vi "KI6221.vi"() -> ()   [LabVIEW 2025] (continued)
                    n1511 = property on="Stop Level" class="DigNum (strict)"() -> ("Value"=w2022:dbl)  [unwired: 2 in, 2 out]
                    n1512 = while {
                      tunnel: w2020 -> [w2061]
                      shift-right: [w2068] -> _
                      shift-left: dbl[] [] -> [w2067]
                      tunnel: w2022 -> [w2066]
                      tunnel: w2008 -> [w2065]
                      i -> [w2058]
                      stop <- w2059 stop-if-true
                      n1513 = Subtract(x=w2065, y=1) -> (x-y=w2057:i32)
                      n1514 = Subtract(x=w2066, y=w2061) -> (x-y=w2063:dbl)
                      n1515 = Divide(x=w2063, y=w2057) -> (x/y=w2062:dbl)
                      n1516 = Multiply(x=w2062, y=w2058) -> (x*y=w2060:dbl)
                      n1517 = Add(x=w2061, y=w2060) -> (x+y=w2056:dbl)
                      n1518 = Insert Into Array(array=w2067, index=w2058, new element=w2056) -> (w2068:dbl[])
                      n1519 = Equal?(x=w2057, y=w2058) -> (x = y?=w2059:bool)
                    }
                    n1520 = while {
                      shift-right: [w2047] -> w2012
                      shift-left: w2011 -> [w2044]
                      shift-right: [w2046] -> w2013
                      shift-left: w2011 -> [w2043]
                      shift-right: [w2045] -> w2014
                      shift-left: w2011 -> [w2042]
                      tunnel: w2010 -> [w2040]
                      tunnel: [w2034] -> _
                      tunnel: w2004 -> [w2036]
                      tunnel: w2009 -> [w2035]
                      tunnel: w2008 -> [w2034]
                      i -> [w2038]
                      stop <- w2039 stop-if-true
                      n1521 = Multiply(x=6, y=w2038) -> (x*y=w2054:i32)
                      n1522 = Add(x=w2040, y=w2054) -> (x+y=w2053:i32)
                      n1523 = Add(x=w2035, y=w2054) -> (x+y=w2052:i32)
                      n1524 = Add(x=5, y=w2054) -> (x+y=w2051:i32)
                      n1525 = Index Array(array=w2036, index (col)=w2053) -> (element=w2050:string[])  [unwired: 1 in]
                      n1526 = Index Array(array=w2036, index (col)=w2052) -> (element=w2049:string[])  [unwired: 1 in]
                      n1527 = Index Array(array=w2036, index (col)=w2051) -> (element=w2048:string[])  [unwired: 1 in]
                      n1528 = Decrement(x=w2034) -> (x-1=w2037:i32)
                      n1529 = Build Array (concatenate)(w2044, w2050) -> (w2047:string[])
                      n1530 = Build Array (concatenate)(w2043, w2049) -> (w2046:string[])
                      n1531 = Build Array (concatenate)(w2042, w2048) -> (w2045:string[])
                      n1532 = Equal?(x=w2037, y=w2038) -> (x = y?=w2039:bool)
                    }
                    n1533 = call "Basic Properties.vi"("Differential Conductance Surface Plot"=w2015, "Int"=w2016, "fast draw"=TRUE) -> ("3D graph out"=w2007:refnum<k7>, "error out"=w2006:errorcluster)  [unwired: 11 in]
                    n1534 = Fract/Exp String To Number(string=w2012) -> (number=w1997:dbl[])  [unwired: 3 in, 1 out]
                    n1535 = To Variant(anything=w1997) -> (Variant=w1999:variant)
                    n1536 = Fract/Exp String To Number(string=w2013) -> (number=w1996:dbl[])  [unwired: 3 in, 1 out]
                    n1537 = To Variant(anything=w1996) -> (Variant=w1998:variant)
                    n1538 = Fract/Exp String To Number(string=w2014) -> (number=w2005:dbl[])  [unwired: 3 in, 1 out]
                    n1539 = To Variant(anything=w2005) -> (Variant=w2000:variant)
                    n1540 = call "Stub 3d Graph-3.vi"("3D graph out"=w2007, "Variant 3"=w2000, "Variant 2"=w1999, "error out 2"=w2006, "Variant"=w1998) -> ("error out"=→"error out 28":errorcluster)
                  }
                  frame True {
                  }
                }
                n1541 = case shown="True" "edit commands STEP SOURCE" {
                  frame False {
                  }
                  frame True {
                    # "HERE WE NEED TO SET THE STEP\nINPUTS TO THE INSTRUMENT \nCOMMANDS ON FILE FOR EDITING."
                    n1542 = property on="Select step source:" class="Ring (strict)"() -> ("Value"=w1987:u16)  [unwired: 2 in, 2 out]
                    n1543 = property on="MASTER DRIVER Array" class="Arr (strict)"() -> ("Value"=w1986:T9)  [unwired: 2 in, 2 out]
                    n1544 = property on="COMM\nTab Control" class="TabCtl (strict)"("Value"=T2."STEP CONFIG" ("COMM\nTab Control")) -> ()  [unwired: 2 in, 2 out]
                    n1545 = Index Array(array=w1986, index=w1987) -> (element=w1985:T14)
                    n1546 = property on="STEP EDIT VAR" class="Bool (strict)"("Value"=TRUE) -> ()  [unwired: 2 in, 2 out]
                    n1547 = Unbundle(w1985) -> ("Numeric"=w1984:i32, "String"=w1983:string, "String 2"=w1982:string, "String 3"=w1981:string, "String 4"=w1980:string, "String 5"=w1979:string, "String 6"=w1978:string, "Numeric 2"=w1977:i32)
                    n1548 = property on="GPIB Address:" class="DigNum (strict)"("Value"=w1984) -> ()  [unwired: 2 in, 2 out]
                    n1549 = property on="INSTRUMENT NAME:" class="Str"("Value"=w1983) -> ()  [unwired: 2 in, 2 out]
                    n1550 = property on="VERIFY:" class="Str"("Value"=w1982) -> ()  [unwired: 2 in, 2 out]
                    n1551 = property on="RESPONSE STRING:" class="Str"("Value"=w1981) -> ()  [unwired: 2 in, 2 out]
                    n1552 = local write "Main Tabs"(T1."General" ("Big Tabs")) -> ()
                    n1553 = property on="CONFIGURE:" class="Str"("Value"=w1980) -> ()  [unwired: 2 in, 2 out]
                    n1554 = property on="GO TO LEVEL:                *NOTE - MUST include <LEVEL>" class="Str"("Value"=w1979) -> ()  [unwired: 2 in, 2 out]
                    n1555 = property on="DEACTIVATE:" class="Str"("Value"=w1978) -> ()  [unwired: 2 in, 2 out]
                    n1556 = property on="DELAY in mS" class="DigNum (strict)"("Value"=w1977) -> ()  [unwired: 2 in, 2 out]
                  }
                }
                n1557 = case shown="True" "DELETE SOURCE" {
                  frame False {
                  }
                  frame True {
                    n1558 = property on="Select step source:" class="Ring (strict)"() -> ("Value"=w1972:u16, "Strings []"=w1974:string[])  [unwired: 2 in, 2 out]
                    n1559 = property on="MASTER DRIVER Array" class="Arr (strict)"() -> ("Value"=w1971:T9)  [unwired: 2 in, 2 out]
                    n1560 = Delete From Array(array=w1974, index=w1972) -> (array with subset deleted=w1975:string[])  [unwired: 1 in, 1 out]
                    n1561 = Decrement(x=w1972) -> (x-1=w1973:u16)
                    n1562 = property on="Select step source:" class="Ring (strict)"("Strings []"=w1975, "Value"=w1973) -> ()  [unwired: 2 in, 2 out]
                    n1563 = Delete From Array(array=w1971, index=w1972) -> (array with subset deleted=w1968:T9)  [unwired: 1 in, 1 out]
                    n1564 = property on="MASTER DRIVER Array" class="Arr (strict)"("Value"=w1968) -> ()  [unwired: 2 in, 2 out]
                    n1565 = property on="Default path" class="Path"() -> ("Value"=w1967:path)  [unwired: 2 in, 2 out]
                    n1566 = Build Path(base path=w1967, name or relative path="stepdriver.cfg" ("file path (dialog if empty)")) -> (appended path=w1965:path)
                    n1567 = Delete(path (use dialog)=w1965) -> (deleted path=w1969:path, error out=→"error out 11":errorcluster)  [unwired: 4 in, 1 out]
                    n1568 = Flatten To String(anything=w1968) -> (data string=w1970:string)  [unwired: 3 in, 2 out]
                    n1569 = call "WriteToFile.vi"("character string"=w1970, "file path (dialog if empty)"=w1969) -> ()  [unwired: 3 in, 1 out]
                  }
                }
                n1570 = property on="Select step source:" class="Ring (strict)"() -> ("Strings []"=w1862:string[])  [unwired: 2 in, 2 out]
                n1571 = Array Size(array=w1862) -> (size(s)=w1861:i32)
                n1572 = Not Equal?(x="Select step source:", y="STEP SOURCE LAST") -> (x != y?=w1855:bool)
                n1573 = Decrement(x=w1861) -> (x-1=w1860:i32)
                n1574 = Equal?(x="Select step source:", y=w1860) -> (x = y?=w1857:bool)
                n1575 = Not(x=w1857) -> (.not. x?=w1856:bool)
                n1576 = And(x=w1856, y=w1855) -> (x .and. y?=w1863:bool)
                n1577 = case shown="True" w1863 {
                  tunnel: "Select step source:" -> [_ w1953]
                  frame False {
                  }
                  frame True {
                    n1578 = property on="MASTER DRIVER Array" class="Arr (strict)"() -> ("Value"=w1954:T9)  [unwired: 2 in, 2 out]
                    n1579 = property on="STEP SOURCE LAST" class="DigNum (strict)"("Value"=w1953) -> ()  [unwired: 2 in, 2 out]
                    n1580 = Index Array(array=w1954, index=w1953) -> (element=w1955:T14)
                    n1581 = Unbundle(w1955) -> ("Numeric"=w1956:i32, "String"=w1957:string, "String 2"=w1958:string, "String 3"=w1959:string, "String 4"=w1960:string, "String 5"=w1961:string, "String 6"=w1962:string, "Numeric 2"=w1963:i32)
                    n1582 = property on="GPIB Address:" class="DigNum (strict)"("Value"=w1956) -> ()  [unwired: 2 in, 2 out]
                    n1583 = property on="INSTRUMENT NAME:" class="Str"("Value"=w1957) -> ()  [unwired: 2 in, 2 out]
                    n1584 = property on="VERIFY:" class="Str"("Value"=w1958) -> ()  [unwired: 2 in, 2 out]
                    n1585 = property on="RESPONSE STRING:" class="Str"("Value"=w1959) -> ()  [unwired: 2 in, 2 out]
                    n1586 = property on="CONFIGURE:" class="Str"("Value"=w1960) -> ()  [unwired: 2 in, 2 out]
                    n1587 = property on="GO TO LEVEL:                *NOTE - MUST include <LEVEL>" class="Str"("Value"=w1961) -> ()  [unwired: 2 in, 2 out]
                    n1588 = property on="DEACTIVATE:" class="Str"("Value"=w1962) -> ()  [unwired: 2 in, 2 out]
                    n1589 = property on="DELAY in mS" class="DigNum (strict)"("Value"=w1963) -> ()  [unwired: 2 in, 2 out]
                  }
                }
                n1590 = case shown="True" w1857 {
                  frame False {
                  }
                  frame True {
                    w1992 = ""
                    w1993 = 20
                    n1591 = property on="STEP EDIT VAR" class="Bool (strict)"("Value"=FALSE ("Visible")) -> ()  [unwired: 2 in, 2 out]
                    n1592 = local write "Main Tabs"(T1."General" ("Big Tabs")) -> ()
                    n1593 = property on="COMM\nTab Control" class="TabCtl (strict)"("Value"=T2."STEP CONFIG" ("COMM\nTab Control")) -> ()  [unwired: 2 in, 2 out]
                    n1594 = property on="GPIB Address:" class="DigNum (strict)"("Value"=w1993) -> ()  [unwired: 2 in, 2 out]
                    n1595 = property on="INSTRUMENT NAME:" class="Str"("Value"=w1992) -> ()  [unwired: 2 in, 2 out]
                    n1596 = property on="VERIFY:" class="Str"("Value"=w1992) -> ()  [unwired: 2 in, 2 out]
                    n1597 = property on="RESPONSE STRING:" class="Str"("Value"=w1992) -> ()  [unwired: 2 in, 2 out]
                    n1598 = property on="CONFIGURE:" class="Str"("Value"=w1992) -> ()  [unwired: 2 in, 2 out]
                    n1599 = property on="GO TO LEVEL:                *NOTE - MUST include <LEVEL>" class="Str"("Value"=w1992) -> ()  [unwired: 2 in, 2 out]
                    n1600 = property on="DEACTIVATE:" class="Str"("Value"=w1992) -> ()  [unwired: 2 in, 2 out]
                    n1601 = property on="DELAY in mS" class="DigNum (strict)"("Value"=w1993) -> ()  [unwired: 2 in, 2 out]
                  }
                }
                n1602 = case shown="0, Default" "I want to control my test in terms of:" {
                  frame 0, Default {
                    w1909 = 105.0 ("y")
                    w1896 = 2
                    # "overlimit\nmultiplier"
                    n1603 = local read "Number of sweep points"() -> (w1914:i32)
                    n1604 = local read "Start Voltage  (Volts)"() -> (w1918:dbl)
                    n1605 = Absolute Value(x=w1918) -> (abs(x)=w1897:dbl)
                    n1606 = local read "Stop Voltage (Volts)"() -> (w1917:dbl)
                    n1607 = Absolute Value(x=w1917) -> (abs(x)=w1898:dbl)
                    n1608 = Greater?(x=w1897, y=w1898) -> (0:w1920:bool)
                    n1609 = Select(t=w1897, s=w1920, f=w1898) -> (s? t:f=w1919:dbl)
                    n1610 = Subtract(x=w1918, y=w1917) -> (x-y=w1915:dbl)
                    n1611 = Absolute Value(x=w1919) -> (abs(x)=w1911:dbl)
                    n1612 = Absolute Value(x=w1915) -> (abs(x)=w1910:dbl)
                    n1613 = Divide(x=w1910, y=w1914) -> (x/y=w1916:dbl)
                    n1614 = Add(x=w1911, y=w1916) -> (x+y=w1913:dbl)
                    n1615 = Multiply(x=w1913, y=1.15) -> (x*y=w1905:dbl)
                    n1616 = Greater?(x=w1905, y=w1909) -> (0:w1908:bool)
                    n1617 = Greater?(x=w1905, y=12.0) -> (0:w1906:bool)
                    n1618 = case shown="False" w1906 {
                      tunnel: [w1934 100.0 ("y")] -> w1899
                      tunnel: w1905 -> [w1933 _]
                      frame False {
                        n1619 = Greater?(x=w1933, y=1.2) -> (0:w1935:bool)
                        n1620 = case shown="False" w1935 {
                          tunnel: [w1938 10.0 ("y")] -> w1934
                          tunnel: w1933 -> [w1937 _]
                          frame False {
                            n1621 = Greater?(x=w1937, y=0.12) -> (0:w1939:bool)
                            n1622 = case shown="False" w1939 {
                              tunnel: [w1942 1.0 ("y")] -> w1938
                              tunnel: w1937 -> [w1941 _]
                              frame False {
                                n1623 = Greater?(x=w1941, y=0.012) -> (0:w1943:bool)
                                n1624 = case shown="False" w1943 {
                                tunnel: [0.01 0.1 ("y")] -> w1942
                                frame False {
                                }
                                frame True {
                                }
                                }
                              }
                              frame True {
                              }
                            }
                          }
                          frame True {
                          }
                        }
                      }
                      frame True {
                      }
                    }
                    n1625 = property on="Voltage Measure Range" class="Ring (strict)"("Disabled"=w1896, "Value"=w1899) -> ()  [unwired: 2 in, 2 out]
                    n1626 = case shown="False" w1908 {
                      tunnel: w1909 -> [_ w1951]
                      tunnel: [w1950 w1951] -> w1904
                      tunnel: w1905 -> [w1950 _]
                      frame False {
                      }
                      frame True {
                      }
                    }
                    n1627 = case shown="False" "Case Constant\n(See Context Help) 5" {
                      tunnel: w1904 -> [w1928 w1932]
                      tunnel: [w1922 w1931] -> w1902
                      frame False {
                        w1921 = 0.1 ("y")
                        w1925 = 100.0 ("y")
                        n1628 = Multiply(x=w1928, y=w1925) -> (x*y=w1927:dbl)
                        n1629 = Round Toward +Infinity(x=w1927) -> (ceil(x): smallest int >= x=w1926:dbl)
                        n1630 = Divide(x=w1926, y=w1925) -> (x/y=w1923:dbl)
                        n1631 = Greater?(x=w1923, y=w1921) -> (0:w1924:bool)
                        n1632 = case shown="False" w1924 {
                          tunnel: [w1929 w1930] -> w1922
                          tunnel: w1923 -> [_ w1930]
                          tunnel: w1921 -> [w1929 _]
                          frame False {
                          }
                          frame True {
                          }
                        }
                      }
                      frame True {
                        n1633 = Round Toward +Infinity(x=w1932) -> (ceil(x): smallest int >= x=w1931:dbl)
                      }
                    }
                    n1634 = Multiply(x=w1902, y=1.2) -> (x*y=w1901:dbl)
                    n1635 = property on="Current Source \nVoltage Compliance (V)" class="DigNum (strict)"("Disabled"=w1896, "Value"=w1901) -> ()  [unwired: 2 in, 2 out]
                  }
                  frame 1 {
                    w1952 = u8 0 ("Disabled")
                    n1636 = property on="Current Source \nVoltage Compliance (V)" class="DigNum (strict)"("Disabled"=w1952) -> ()  [unwired: 2 in, 2 out]
                    n1637 = property on="Voltage Measure Range" class="Ring (strict)"("Disabled"=w1952) -> ()  [unwired: 2 in, 2 out]
                  }
                }
              }
              frame "Pulsed IV Measurements" {
                # "Fliter visible..."
                # "PULSE CONTROLS NOT DIRECTLY LINKED."
                # "CLEAR DATA from sheet and graph"
                # "SAVE DATA to file"
                # "Update Pulse TABS"
                # "UPDATE GRAPH AXIS WHEN SELECTIONS ARE CHANGED"
                # "ENABLE PULSE COUNT ON INF OFF SETTING"
                n1638 = case shown="0, Default" "Pulse Mode:" {
                  tunnel: [enum32{"DIAGRAM 2", "DIAGRAM"}."DIAGRAM 2" ("PULSE HELP TABS") enum32{"DIAGRAM 2", "DIAGRAM"}."DIAGRAM" ("PULSE HELP TABS")] -> w3061
                  frame 0, Default {
                  }
                  frame 1 {
                  }
                }
                n1639 = local write "PULSE SWEEP OR LEVEL TABS"("Pulse Mode:") -> ()
                n1640 = Boolean To (0,1)(Boolean="INFINITE REPEAT PULSE CYCLES") -> (0, 1=w3077:i16)
                n1641 = Multiply(x=w3077, y=i16 2) -> (x*y=w3076:i16)
                n1642 = property on="Number of Readings" class="DigNum (strict)"("Disabled"=w3076) -> ()  [unwired: 2 in, 2 out]
                n1643 = local write "PULSE HELP TABS"(w3061) -> ()
                n1644 = case shown="True" "PULSE SAVE DATA" {
                  frame False {
                  }
                  frame True {
                    n1645 = File Dialog(4:"KI Data files" ("pattern label"), 5:"Save As" ("button label"), 6:"*.kdf" ("pattern label")) -> (1:w3633:bool, 3:w3632:path)  [unwired: 4 in, 2 out]
                    n1646 = case shown="False" w3633 {
                      tunnel: w3632 -> [w3637 _]
                      frame False {
                        w3641 = "%s" ("format string")
                        n1647 = property on="PULSE DATA SHEET" class="Tbl (strict)"() -> ("Column Header Strings[]"=w3642:string[], "Value"=w3643:string[][])  [unwired: 2 in, 2 out]
                        n1648 = Array To Spreadsheet String(array=w3643, 3:w3641) -> (spreadsheet string=w3639:string)  [unwired: 1 in]
                        n1649 = Array To Spreadsheet String(array=w3642, 3:w3641) -> (spreadsheet string=w3640:string)  [unwired: 1 in]
                        n1650 = Concatenate Strings(w3640, w3639) -> (w3638:string)
                        n1651 = call "WriteToFile.vi"("character string"=w3638, "file path (dialog if empty)"=w3637) -> ()  [unwired: 3 in, 1 out]
                      }
                      frame True {
                      }
                    }
                  }
                }
                n1652 = case shown="True" "RUN PULSE" {
                  frame False {
                  }
                  frame True {
                    w3103 = FALSE
                    w3101 = TRUE
                    w3130 = "%s" ("format string")
                    w3111 = 0
                    w3113 = u16 2 ("x")
                    # "SETUP FOR TEST RUN. INIT controls."
                    # "RESET ENABLES FOR \nNEW TEST RUN."
                    n1653 = property on="ABORT PULSE" class="Bool (strict)"("Value"=FALSE, "Disabled"=u16 0 ("x")) -> (error out=w3137:errorcluster)  [unwired: 2 in, 1 out]
                    n1654 = property on="Main Tabs" class="TabCtl (strict)"("Page Selector Visible"=w3103) -> (error out=w3104:errorcluster)  [unwired: 2 in, 1 out]
                    n1655 = property on="Advanced Operation Tab" class="TabCtl (strict)"(error in=w3104, "Page Selector Visible"=w3103) -> (error out=w3114:errorcluster)  [unwired: 1 in, 1 out]
                    n1656 = local read "Current Test File:"() -> (w3105:path)
                    n1657 = Equal?(x=w3105, y=path "") -> (x = y?=w3119:bool)
                    n1658 = case shown="True" w3119 {
                      tunnel: w3105 -> [w3151 _]
                      tunnel: [w3146 w3152] -> w3118
                      frame False {
                        n1659 = Path To String(path=w3151) -> (string=w3149:string)
                        n1660 = Search/Split String(string=w3149, search string/char (-)=".") -> (substring before match=w3148:string)  [unwired: 1 in, 2 out]
                        n1661 = Concatenate Strings(w3148, "_pulsedata.kdf" ("search string/char (-)")) -> (w3145:string)
                        n1662 = String To Path(string=w3145) -> (path=w3146:path)
                      }
                      frame True {
                        n1663 = property on="Default path" class="Path"() -> ("Value"=w3154:path)  [unwired: 2 in, 2 out]
                        n1664 = Build Path(base path=w3154, name or relative path="DefaultTestFile_pulsedata.cfg" ("file path (dialog if empty)")) -> (appended path=w3152:path)
                      }
                    }
                    n1665 = property on="RUN PULSE" class="Bool"(error in=w3114, "Disabled"=w3113) -> (error out=w3116:errorcluster)  [unwired: 1 in, 1 out]
                    n1666 = invoke on="PULSE DATA SHEET" class="Table" method="Reinit To Default"(error in=w3116) -> (error out=w3108:errorcluster)  [unwired: 2 in, 2 out]
                    n1667 = invoke on="Pulsed IV Graph" class="XYGraph (strict)" method="Reinit To Default"(error in=w3108) -> (error out=w3107:errorcluster)  [unwired: 2 in, 2 out]
                    n1668 = property on="DEMO MODE" class="Bool (strict)"(error in=w3107) -> ("Value"=w3144:bool)  [unwired: 1 in, 2 out]
                    n1669 = property on="X Axis:" class="Ring (strict)"("Disabled"=w3113) -> ("Value"=w3140:u16, "Strings []"=w3143:string[])  [unwired: 2 in, 2 out]
                    n1670 = Index Array(array=w3143, index=w3140) -> (element=w3110:string)
                    n1671 = property on="Y Axis:" class="Ring (strict)"("Disabled"=w3113) -> ("Value"=w3141:u16, "Strings []"=w3142:string[])  [unwired: 2 in, 2 out]
                    n1672 = call <vilib>:"Read Lines From File.vi"("convert eol? (no:F)"=TRUE, "file path (dialog if empty)"=w3118, "number of lines (all:-1)"=-1) -> ("line string"=w3128:string)  [unwired: 3 in, 3 out]
                    n1673 = Match Pattern(string=w3128, regular expression="\n") -> (before substring=w3126:string, match substring=w3125:string, after substring=w3123:string)  [unwired: 1 in, 1 out]
                    n1674 = Index Array(array=w3142, index=w3141) -> (element=w3109:string)
                    n1675 = property on="Pulsed IV Graph" class="XYGraph (strict)"("X Scale.Name Label.Text"=w3110, "Y Scale.Name Label.Text"=w3109) -> ()  [unwired: 2 in, 2 out]
                    n1676 = Concatenate Strings(w3126, w3125) -> (w3124:string)
                    n1677 = Spreadsheet String To Array(format string=w3130, spreadsheet string=w3123, array type (2D Dbl)=string[][] []) -> (array=w3117:string[][])  [unwired: 1 in]
                    n1678 = Spreadsheet String To Array(format string=w3130, spreadsheet string=w3124, array type (2D Dbl)=string[] []) -> ()  [unwired: 1 in, 1 out]
                    n1679 = case shown="False" w3144 {
                      tunnel: w3117 -> [_ w3590]
                      tunnel: w3141 -> [_ w3588]
                      tunnel: w3140 -> [_ w3589]
                      tunnel: w3137 -> [w3176 w3596]
                      tunnel: [w3176 w3596] -> w3136
                      tunnel: [w3175 w3587] -> w3133
                      frame False {
                        # "PULSE MODE CONTROL\nCHECKS - OK TO \nCONTINUE WITH RUN?"
                        n1680 = property on="Select the nanovoltmeter model number:" class="Ring (strict)"() -> ("Value"=w3181:u16)  [unwired: 2 in, 2 out]
                        n1681 = property on="Start Pulse Level (Amps)" class="DigNum (strict)"() -> ("Value"=w3191:dbl)  [unwired: 2 in, 2 out]
                        n1682 = property on="Stop Pulse Level (Amps)" class="DigNum (strict)"() -> ("Value"=w3190:dbl)  [unwired: 2 in, 2 out]
                        n1683 = property on="Pulse Mode:" class="Ring (strict)"() -> ("Value"=w3192:u16)  [unwired: 2 in, 2 out]
                        n1684 = property on="Sweep Type" class="Ring (strict)"() -> ("Value"=w3185:u16)  [unwired: 2 in, 2 out]
                        n1685 = property on="Select the current source model number:" class="Ring (strict)"() -> ("Value"=w3174:u16)  [unwired: 2 in, 2 out]
                        n1686 = Equal?(x=w3181, y=3) -> (x = y?=w3178:bool)
                        n1687 = Equal?(x=w3174, y=2) -> (x = y?=w3155:bool)
                        n1688 = property on="Pulse Width (mS)" class="DigNum (strict)"() -> ("Value"=w3173:dbl)  [unwired: 2 in, 2 out]
                        n1689 = Not Equal To 0?(x=w3192) -> (x != 0?=w3186:bool)
                        n1690 = Greater Than 0?(x=w3191) -> (x > 0?=w3189:bool)
                        n1691 = property on="Delay - pulse settle time in mS" class="DigNum (strict)"() -> ("Value"=w3159:dbl)  [unwired: 2 in, 2 out]
                        n1692 = Less?(x=w3159, y=0.5) -> (x < y?=w3168:bool)
                        n1693 = And(x=w3178, y=w3155) -> (x .and. y?=w3177:bool)
                        n1694 = Equal To 0?(x=w3185) -> (x = 0?=w3184:bool)
                        n1695 = Less?(x=w3159, y=0.055) -> (x < y?=w3164:bool)
                        n1696 = Greater Than 0?(x=w3190) -> (x > 0?=w3188:bool)
                        n1697 = And(x=w3189, y=w3188) -> (x .and. y?=w3187:bool)
                        n1698 = property on="Voltage Measure Range" class="Ring (strict)"() -> ("Value"=w3156:dbl)  [unwired: 2 in, 2 out]
                        n1699 = Equal?(x=100.0, y=w3156) -> (x = y?=w3166:bool)
                        n1700 = And(x=w3168, y=w3166) -> (x .and. y?=w3169:bool)
                        n1701 = Add(x=0.034, y=w3159) -> (x+y=w3171:dbl)
                        n1702 = Greater Or Equal?(x=w3173, y=w3171) -> (x >= y?=w3172:bool)
                        n1703 = Compound Arithmetic op=OR(w3186, w3187, w3184) -> (w3182:bool)
                        n1704 = Equal?(x=0.01, y=w3156) -> (x = y?=w3162:bool)
                        n1705 = And(x=w3164, y=w3162) -> (x .and. y?=w3160:bool)
                        n1706 = Or(x=w3169, y=w3160) -> (x .or. y?=w3158:bool)
                        n1707 = case shown="True" w3158 {
                          tunnel: [TRUE ("OK") w3194] -> w3157
                          frame False {
                          }
                          frame True {
                            # "SEND WARNING"
                            n1708 = call "Pulse delay warning"() -> ("OK"=w3194:bool)  [unwired: 10 in, 1 out]
                          }
                        }
                        n1709 = Compound Arithmetic op=AND(w3182, w3177, w3172, w3157) -> (w3183:bool)
                        n1710 = case shown="False" w3183 {
                          tunnel: w3182 -> [w3198 _]
                          tunnel: w3177 -> [w3197 _]
                          tunnel: [FALSE w3209] -> w3175
                          tunnel: w3172 -> [w3195 _]
                          tunnel: w3156 -> [_ w3208]
                          frame False {
                            n1711 = case shown="False" w3195 {
                              frame False {
                                n1712 = One Button Dialog(message="For Pulsed IV measurements the pulse width must be greater than or equal to\nthe delay (settling time) plus 34 us for the measurement. Please correct the settings.") -> (true=w3199:bool)  [unwired: 1 in]
                                n1713 = case shown="False" w3199 {
                                frame False {
                                }
                                frame True, Default {
                                n1714 = property on="Delay - pulse settle time in mS" class="DigNum (strict)"("Key Focus"=TRUE) -> ()  [unwired: 2 in, 2 out]
                                }
                                }
                              }
                              frame True {
                              }
                            }
                            n1715 = case shown="False" w3197 {
                              frame False {
                                n1716 = One Button Dialog(message="Taking pulsed IV measurements requires both a Model 6221 current\nsource and a Model 2182A nanovoltmeter connected to the bus and \nconfigured in the instrument communication panel.") -> (true=w3202:bool)  [unwired: 1 in]
                                n1717 = case shown="False" w3202 {
                                frame False {
                                }
                                frame True, Default {
                                }
                                }
                              }
                              frame True {
                              }
                            }
                            n1718 = case shown="False" w3198 {
                              frame False {
                                n1719 = One Button Dialog(message="To run a test with a logarithmic pulse sweep, both start and stop\npulse values must be positive. Change a value, then click RUN again.") -> (true=w3204:bool)  [unwired: 1 in]
                                n1720 = case shown="True" w3204 {
                                frame False {
                                }
                                frame True, Default {
                                n1721 = property on="Start Pulse Level (Amps)" class="DigNum (strict)"("Key Focus"=TRUE) -> ()  [unwired: 2 in, 2 out]
                                }
                                }
                              }
                              frame True {
                              }
                            }
                          }
                          frame True {
                            (unwired) "Initiating Test. Make certain device is correctly connected\nto the instruments, then click OK. "
                            # "ACTUAL DATA \nCOMMUNICATION"
                            n1722 = property on="X Axis:" class="Ring (strict)"() -> ("Value"=w3211:u16)  [unwired: 2 in, 2 out]
                            n1723 = property on="Y Axis:" class="Ring (strict)"() -> ("Value"=w3210:u16)  [unwired: 2 in, 2 out]
                            n1724 = case shown="True" "Case Constant\n(See Context Help) 6" {
                              tunnel: [FALSE w3219] -> w3209
                              tunnel: w3211 -> [_ w3223]
                              tunnel: w3210 -> [_ w3222]
                              tunnel: w3208 -> [_ w3220]
                              frame False {
                              }
                              frame True {
                                # "TEST MODEL NUMBER AT VISA \nRESOURCE..."
                                # "no NV"
                                # "NOT 6221"
                                n1725 = property on="6220 VISA" class="VISAName"() -> ("Value"=w3218:refnum<visa-resource-name>)  [unwired: 2 in, 2 out]
                                n1726 = property on="GPIB Array" class="Arr (strict)"() -> ("Value"=w3217:string[])  [unwired: 2 in, 2 out]
                                n1727 = call "VISAreadWrite.vi"("GPIB INDEX Array"=i32[] [0, 14], "GPIB ARRAY"=w3217, "VISA REFERENCE"=w3218) -> ("error out 15"=→"error out 17":errorcluster, "Read Buffer Array"=w3229:string[])  [unwired: 1 in]
                                n1728 = Index Array(array=w3229, index=1) -> (element=w3234:string)
                                n1729 = Match Pattern(string=w3234, regular expression="MODEL 6221") -> (offset past match=w3226:i32)  [unwired: 1 in, 3 out]
                                n1730 = Equal?(x=w3226, y=-1) -> (x = y?=w3224:bool)
                                n1731 = Index Array(array=w3229, index=5) -> (element=w3228:string)
                                n1732 = Decimal String To Number(string=w3228) -> (number=w3227:i32)  [unwired: 2 in, 1 out]
                                n1733 = Equal To 0?(x=w3227) -> (x = 0?=w3225:bool)
                                n1734 = Or(x=w3225, y=w3224) -> (x .or. y?=w3214:bool)
                                n1735 = case shown="False" w3214 {
                                tunnel: w3225 -> [_ w3585]
                                tunnel: w3224 -> [_ w3583]
                                tunnel: w3217 -> [w3361 _]
                                tunnel: w3218 -> [w3315 _]
                                tunnel: w3223 -> [w3310 _]
                                tunnel: w3222 -> [w3338 _]
                                tunnel: w3220 -> [w3296 _]
                                tunnel: [TRUE FALSE] -> w3213
                                frame False {
                                # "SWEEP RANGE FOR LOG - AUTO\ndc SWEEPS TOO.\nif off value < 2% of Max current value of pulse \nOR < 4 pA then do power..."
                                # "special pulse sweep delay fix\nround(NPLC*INC-6)/1000 = delay"
                                # "type"
                                # "count"
                                # "state"
                                # "TEST FOR ALL ZERO\nMEASUREMENTS FROM\nRANGE ERROR - DISP\nMessage..."
                                # "UPDATE SCPI STRINGS THEN LOAD THEM TO THE INSTRUMENT."
                                # "CREATE SCPI STRINGS FROM CONTROLS"
                                # "Check for data in buffer... when you get some, place it in data sheet and graph. REPEAT until all data is collected."
                                # "FIX SOURCE CURRENT"
                                n1736 = property on="Pulse Mode:" class="Ring (strict)"() -> ("Value"=w3264:u16)  [unwired: 2 in, 2 out]
                                n1737 = property on="Interval between Pulses (NPLC)" class="DigNum (strict)"() -> ("Value"=w3272:dbl)  [unwired: 2 in, 2 out]
                                n1738 = property on="Pulse Width (mS)" class="DigNum (strict)"() -> ("Value"=w3302:dbl)  [unwired: 2 in, 2 out]
                                n1739 = Not Equal To 0?(x="PULSE FILTER") -> (x != 0?=w3286:bool)
                                n1740 = property on="Number of Readings" class="DigNum (strict)"() -> ("Value"=w3321:i32)  [unwired: 2 in, 2 out]
                                n1741 = property on="INFINITE REPEAT PULSE CYCLES" class="Bool (strict)"() -> ("Value"=w3360:bool)  [unwired: 2 in, 2 out]
                                n1742 = local read "Pulse Filter Count"() -> (w3292:i32)
                                n1743 = case shown="2" "PULSE FILTER" {
                                tunnel: ["MOV" "MOV" "REP"] -> w3291
                                frame 0, Default {
                                }
                                frame 1 {
                                }
                                frame 2 {
                                }
                                }
                                n1744 = property on="Start Pulse Level (Amps)" class="DigNum (strict)"() -> ("Value"=w3263:dbl)  [unwired: 2 in, 2 out]
                                n1745 = property on="Stop Pulse Level (Amps)" class="DigNum (strict)"() -> ("Value"=w3262:dbl)  [unwired: 2 in, 2 out]
                                n1746 = property on="Pulse Level (Amps)" class="DigNum (strict)"() -> ("Value"=w3261:dbl)  [unwired: 2 in, 2 out]
                                n1747 = property on="Number of Pulses" class="DigNum (strict)"() -> ("Value"=w3319:i32)  [unwired: 2 in, 2 out]
                                n1748 = property on="Sweep Type" class="Ring (strict)"() -> ("Value"=w3249:u16)  [unwired: 2 in, 2 out]
                                n1749 = Equal?(x=w3249, y=u16 1) -> (x = y?=w3285:bool)
                                n1750 = property on="Pulse Off Level (Amps)" class="DigNum (strict)"() -> ("Value"=w3256:dbl)  [unwired: 2 in, 2 out]
                                n1751 = And(x=w3286, y=w3285) -> (x .and. y?=w3284:bool)
                                n1752 = property on="Delay - pulse settle time in mS" class="DigNum (strict)"() -> ("Value"=w3304:dbl)  [unwired: 2 in, 2 out]
                                n1753 = case shown="False" w3284 {
                                tunnel: ["0" "1"] -> w3289
                                frame False {
                                }
                                frame True {
                                }
                                }
                                n1754 = Number To Decimal String(number=w3272) -> (decimal integer string=w3346:string)  [unwired: 1 in]
                                n1755 = Negate(x=w3256) -> (-x=w3330:dbl)
                                n1756 = Divide(x=w3302, y=1000.0) -> (x/y=w3301:dbl)
                                n1757 = Divide(x=w3304, y=1000.0) -> (x/y=w3300:dbl)
                                n1758 = Number To Decimal String(number=w3292) -> (decimal integer string=w3290:string)  [unwired: 1 in]
                                n1759 = Number To Exponential String(number=w3261) -> (E-format string=w3349:string)  [unwired: 3 in]
                                n1760 = case shown="1" w3264 {
                                tunnel: ["1" "0"] -> w3329
                                tunnel: w3321 -> [_ w3576]
                                tunnel: [w3574 w3576] -> w3320
                                tunnel: w3319 -> [w3574 _]
                                frame 0, Default {
                                }
                                frame 1 {
                                }
                                }
                                n1761 = Equal?(x=w3330, y=w3261) -> (x = y?=w3316:bool)
                                n1762 = property on="Current Source \nVoltage Compliance (V)" class="DigNum (strict)"() -> ("Value"=w3340:dbl)  [unwired: 2 in, 2 out]
                                n1763 = Number To Exponential String(number=w3256) -> (E-format string=w3348:string)  [unwired: 3 in]
                                n1764 = Number To Exponential String(number=w3301) -> (E-format string=w3345:string)  [unwired: 3 in]
                                n1765 = Number To Exponential String(number=w3300) -> (E-format string=w3343:string)  [unwired: 3 in]
                                n1766 = Number To Exponential String(number=w3340) -> (E-format string=w3328:string)  [unwired: 3 in]
                                n1767 = case shown="1" w3249 {
                                tunnel: ["BEST" "AUTO"] -> w3248
                                frame 0, Default {
                                }
                                frame 1 {
                                }
                                }
                                n1768 = Decrement(x=w3319) -> (x-1=w3318:i32)
                                n1769 = case shown="False" w3360 {
                                tunnel: [w3579 "INF"] -> w3347
                                tunnel: w3320 -> [w3578 _]
                                tunnel: [w3578 0 ("Value")] -> w3311
                                frame False {
                                n1770 = Number To Decimal String(number=w3578) -> (decimal integer string=w3579:string)  [unwired: 1 in]
                                }
                                frame True {
                                }
                                }
                                n1771 = local read "INCREMENT"() -> (w3271:dbl)
                                n1772 = Multiply(x=w3272, y=w3271) -> (x*y=w3279:dbl)
                                n1773 = Divide(x=w3302, y=w3279) -> (x/y=w3305:dbl)
                                n1774 = case shown="1" w3249 {
                                tunnel: ["LIN" "LOG"] -> w3323
                                frame 0, Default {
                                }
                                frame 1 {
                                }
                                }
                                n1775 = Number To Exponential String(number=w3296) -> (E-format string=w3344:string)  [unwired: 3 in]
                                n1776 = Number To Decimal String(number="Number of Pulse Off Measurements") -> (decimal integer string=w3276:string)  [unwired: 1 in]
                                n1777 = Number To Exponential String(number=w3263) -> (E-format string=w3327:string)  [unwired: 3 in]
                                n1778 = Number To Exponential String(number=w3262) -> (E-format string=w3326:string)  [unwired: 3 in]
                                n1779 = Subtract(x=w3262, y=w3263) -> (x-y=w3322:dbl)
                                n1780 = Multiply(x=w3272, y=w3271) -> (x*y=w3270:dbl)
                                n1781 = Divide(x=w3322, y=w3318) -> (x/y=w3274:dbl)
                                n1782 = Number To Exponential String(number=w3274) -> (E-format string=w3325:string)  [unwired: 3 in]
                                n1783 = Subtract(x=w3270, y=6.0) -> (x-y=w3268:dbl)
                                n1784 = Round To Nearest(number=w3268) -> (nearest integer value=w3246:dbl)
                                n1785 = Insert Into Array(array=string[] [] ("Replace Array"), new element=w3349) -> (w3358:string[])  [unwired: 1 in]
                                n1786 = Equal?(x=w3246, y=77.0) -> (x = y?=w3247:bool)
                                n1787 = Insert Into Array(array=w3358, new element=w3348) -> (w3357:string[])  [unwired: 1 in]
                                n1788 = case shown="0, Default" w3264 {
                                tunnel: w3263 -> [w3372 _]
                                tunnel: w3262 -> [w3371 _]
                                tunnel: w3261 -> [_ w3374]
                                tunnel: [w3367 w3373] -> w3254
                                frame 0, Default {
                                n1789 = Absolute Value(x=w3372) -> (abs(x)=w3370:dbl)
                                n1790 = Absolute Value(x=w3371) -> (abs(x)=w3369:dbl)
                                n1791 = Greater?(x=w3370, y=w3369) -> (0:w3368:bool)
                                n1792 = Select(t=w3370, s=w3368, f=w3369) -> (s? t:f=w3367:dbl)
                                }
                                frame 1 {
                                n1793 = Absolute Value(x=w3374) -> (abs(x)=w3373:dbl)
                                }
                                }
                                n1794 = case shown="True" w3247 {
                                tunnel: w3246 -> [w3363 _]
                                tunnel: [w3363 1.0] -> w3244
                                frame False {
                                }
                                frame True {
                                }
                                }
                                n1795 = Insert Into Array(array=w3357, new element=w3347) -> (w3356:string[])  [unwired: 1 in]
                                n1796 = Insert Into Array(array=w3356, new element=w3327) -> (w3355:string[])  [unwired: 1 in]
                                n1797 = Insert Into Array(array=w3355, new element=w3346) -> (w3354:string[])  [unwired: 1 in]
                                n1798 = Insert Into Array(array=w3354, new element=w3345) -> (w3341:string[])  [unwired: 1 in]
                                n1799 = Insert Into Array(array=w3341, new element=w3328) -> (w3353:string[])  [unwired: 1 in]
                                n1800 = Insert Into Array(array=w3353, new element=w3344) -> (w3352:string[])  [unwired: 1 in]
                                n1801 = Insert Into Array(array=w3352, new element=w3343) -> (w3351:string[])  [unwired: 1 in]
                                n1802 = Insert Into Array(array=w3351, new element=w3329) -> (w3350:string[])  [unwired: 1 in]
                                n1803 = Insert Into Array(array=w3350, new element=w3325) -> (w3339:string[])  [unwired: 1 in]
                                n1804 = Insert Into Array(array=w3339, new element=w3326) -> (w3324:string[])  [unwired: 1 in]
                                n1805 = local read "Setup String"() -> (w3298:string)
                                n1806 = Add(x=u16 3, y=w3338) -> (x+y=w3308:u16)
                                n1807 = Divide(x=w3244, y=1000.0) -> (x/y=w3266:dbl)
                                n1808 = Insert Into Array(array=w3324, new element=w3323) -> (w3297:string[])  [unwired: 1 in]
                                n1809 = Number To Exponential String(number=w3266) -> (E-format string=w3265:string)  [unwired: 3 in]
                                n1810 = Absolute Value(x=w3256) -> (abs(x)=w3252:dbl)
                                n1811 = Less?(x=w3254, y=4e-12) -> (x < y?=w3255:bool)
                                n1812 = Divide(x=w3252, y=w3254) -> (x/y=w3259:dbl)
                                n1813 = Less?(x=w3259, y=0.02) -> (x < y?=w3257:bool)
                                n1814 = Or(x=w3257, y=w3255) -> (x .or. y?=w3258:bool)
                                n1815 = Insert Into Array(array=w3297, new element=w3298) -> (w3293:string[])  [unwired: 1 in]
                                n1816 = Insert Into Array(array=w3293, new element=w3289) -> (w3295:string[])  [unwired: 1 in]
                                n1817 = Insert Into Array(array=w3295, new element=w3290) -> (w3294:string[])  [unwired: 1 in]
                                n1818 = Insert Into Array(array=w3294, new element=w3291) -> (w3275:string[])  [unwired: 1 in]
                                n1819 = Insert Into Array(array=w3275, new element=w3276) -> (w3273:string[])  [unwired: 1 in]
                                n1820 = Insert Into Array(array=w3273, new element=w3265) -> (w3251:string[])  [unwired: 1 in]
                                n1821 = Insert Into Array(array=w3251, new element=w3248) -> (w3250:string[])  [unwired: 1 in]
                                n1822 = call "VisaVarReplace.vi"("Replace Array"=w3250, "Search Array"=string[] ["<PULSEHIGH>", "<PULSEOFF>", "<PULSECOUNT>", "<PULSESWEEPSTART>", "<PULSEINTERVAL>", "<PULSEWIDTH>", "<PULSECOMP>", "<PULSEVOLTRANGE>", "<PULSEDELAY>", "<PULSESWEEPSTATE>", "<PULSESWEEPSTEP>", "<PULSESWEEPSTOP>", "<PULSESWEEPSPACING>", "<SETUPSTRING>", "<PULSEFILTERSTATE>", "<PULSEFILTERCOUNT>", "<PULSEFILTERTYPE>", "<PULSELOWMEAS>", "<PULSESWEEPINT>", "<PULSESWEEPRANGE>"], "GPIB Array"=w3361) -> ("GPIB Array OUT"=w3313:string[])
                                n1823 = call "VISAreadWrite.vi"("GPIB INDEX Array"=i32[] [20], "GPIB ARRAY"=w3313, "VISA REFERENCE"=w3315) -> ("error out 15"=w3309:errorcluster)  [unwired: 1 in, 1 out]
                                n1824 = case shown="No Error" w3309 {
                                tunnel: w3315 -> [w3393 w3568]
                                tunnel: w3313 -> [w3392 w3569]
                                tunnel: w3311 -> [w3391 _]
                                tunnel: dbl[] [] -> [w3390 _]
                                tunnel: string[][] [] -> [w3389 _]
                                tunnel: w3310 -> [w3388 _]
                                tunnel: w3308 -> [w3387 _]
                                tunnel: [w3385 string[][] [["", "", "", "1", "3"], ["", "", "", "", "1"], ["", "", "", "", "2"], ["", "", "", "1", ""]]] -> w3307
                                tunnel: w3316 -> [w3386 _]
                                tunnel: 0.0 -> [w3384 _]
                                tunnel: w3305 -> [w3383 _]
                                tunnel: w3256 -> [w3382 _]
                                tunnel: w3258 -> [w3381 _]
                                tunnel: w3256 -> [w3380 _]
                                frame No Error {
                                n1825 = while {
                                tunnel: w3393 -> [w3410]
                                tunnel: w3392 -> [w3409]
                                tunnel: w3391 -> [w3408]
                                tunnel: w3390 -> [w3406]
                                tunnel: w3388 -> [w3404]
                                tunnel: w3387 -> [w3403]
                                tunnel: w3386 -> [w3402]
                                shift-right: [w3401] -> w3385
                                shift-left: w3389 -> [w3405]
                                shift-right: [w3400] -> _
                                shift-left: w3384 -> [w3399]
                                tunnel: w3383 -> [w3397]
                                tunnel: w3382 -> [w3396]
                                tunnel: w3381 -> [w3395]
                                tunnel: w3380 -> [w3394]
                                stop <- w3407 stop-if-true
                                n1826 = case shown="False" "ABORT PULSE" {
                                tunnel: w3410 -> [w3430 _]
                                tunnel: w3409 -> [w3429 _]
                                tunnel: w3408 -> [w3427 _]
                                tunnel: [w3426 w3566] -> w3407
                                tunnel: w3406 -> [w3425 _]
                                tunnel: w3405 -> [w3424 _]
                                tunnel: [w3423 string[][] [["", "", "", "1", "0"], ["", "", "", "", "2"], ["", "", "", "", ""], ["", "", "", "1", ""], ["", "", "", "", "1"]]] -> w3401
                                tunnel: w3404 -> [w3422 _]
                                tunnel: w3403 -> [w3421 _]
                                tunnel: w3402 -> [w3418 _]
                                tunnel: "ABORT PULSE" -> [w3417 w3566]
                                tunnel: [w3416 w3564] -> w3400
                                tunnel: w3399 -> [w3415 w3564]
                                tunnel: w3397 -> [w3414 _]
                                tunnel: w3396 -> [w3413 _]
                                tunnel: w3395 -> [w3412 _]
                                tunnel: w3394 -> [w3411 _]
                                frame False {
                                n1827 = case shown="True" w3419 {
                                tunnel: w3428 -> [_ w3514]
                                tunnel: w3427 -> [_ w3511]
                                tunnel: [FALSE w3510] -> w3426
                                tunnel: w3425 -> [_ w3508]
                                tunnel: w3424 -> [_ w3487]
                                tunnel: [string[][] [["", "", "", ""], ["", "", "", ""], ["", "", "", ""], ["", "", "", "1"]] w3504] -> w3423
                                tunnel: w3422 -> [_ w3503]
                                tunnel: w3421 -> [_ w3502]
                                tunnel: w3420 -> [_ w3495]
                                tunnel: w3418 -> [_ w3494]
                                tunnel: w3417 -> [_ w3493]
                                tunnel: [w3477 w3485] -> w3416
                                tunnel: w3415 -> [w3477 _]
                                tunnel: w3414 -> [_ w3483]
                                tunnel: w3413 -> [_ w3482]
                                tunnel: w3412 -> [_ w3481]
                                tunnel: w3411 -> [_ w3480]
                                frame False {
                                }
                                frame True {
                                n1828 = Decrement(x=w3511) -> (x-1=w3492:i32)
                                n1829 = Bundle(0, 0) -> (w3491:cluster{i32, i32})  [unwired: 1 in]
                                n1830 = Spreadsheet String To Array(delimiter (Tab)=",", format string="%e", spreadsheet string=w3495, array type (2D Dbl)=w3508) -> (array=w3507:dbl[])
                                n1831 = while {
                                tunnel: w3507 -> [w3540]
                                tunnel: [w3539] -> w3486
                                tunnel: w3494 -> [_]
                                shift-right: [w3538] -> w3488
                                shift-left: string[][] [] -> [w3532]
                                tunnel: w3483 -> [w3524]
                                tunnel: w3482 -> [w3519]
                                tunnel: w3481 -> [w3518]
                                tunnel: w3480 -> [w3515]
                                i -> [w3537]
                                stop <- w3552 stop-if-true
                                w3531 = "," ("delimiter (Tab)")
                                n1832 = Array Size(array=w3532) -> (size(s)=w3535:i32[])
                                n1833 = Index Array(array=w3535, index=0) -> (element=w3533:i32)
                                n1834 = Multiply(x=4, y=w3533) -> (x*y=w3555:i32)
                                n1835 = Index Array(array=w3540, index=w3555) -> (element=w3526:dbl)
                                n1836 = Increment(x=w3555) -> (x+1=w3553:i32)
                                n1837 = Index Array(array=w3540, index=w3553) -> (element=w3530:dbl)
                                n1838 = Increment(x=w3553) -> (x+1=w3554:i32)
                                n1839 = Index Array(array=w3540, index=w3554) -> (element=w3516:dbl)
                                n1840 = Subtract(x=w3516, y=w3515) -> (x-y=w3517:dbl)
                                n1841 = Multiply(x=w3526, y=w3517) -> (x*y=w3525:dbl)
                                n1842 = Multiply(x=w3525, y=w3524) -> (x*y=w3523:dbl)
                                n1843 = case shown="True" w3518 {
                                tunnel: [w3557 w3561] -> w3529
                                tunnel: [w3557 w3560] -> w3528
                                tunnel: w3525 -> [_ w3559]
                                tunnel: w3523 -> [_ w3558]
                                frame False {
                                w3557 = "" ("delimiter (Tab)")
                                }
                                frame True {
                                n1844 = Number To Engineering String(4:w3559) -> (0:w3560:string)  [unwired: 3 in]
                                n1845 = Number To Engineering String(4:w3558) -> (0:w3561:string)  [unwired: 3 in]
                                }
                                }
                                n1846 = Subtract(x=w3516, y=w3519) -> (x-y=w3521:dbl)
                                n1847 = Divide(x=w3526, y=w3521) -> (x/y=w3520:dbl)
                                n1848 = Reciprocal(x=w3520) -> (1/x=w3522:dbl)
                                n1849 = Increment(x=w3554) -> (x+1=w3550:i32)
                                n1850 = Array Size(array=w3540) -> (size(s)=w3536:i32)
                                n1851 = Index Array(array=w3540, index=w3550) -> (element=w3539:dbl)
                                n1852 = Increment(x=w3550) -> (x+1=w3551:i32)
                                n1853 = Number To Engineering String(4:w3520) -> (0:w3542:string)  [unwired: 3 in]
                                n1854 = Number To Engineering String(4:w3526) -> (0:w3541:string)  [unwired: 3 in]
                                n1855 = Number To Engineering String(4:w3530) -> (0:w3543:string)  [unwired: 3 in]
                                n1856 = Number To Engineering String(4:w3516) -> (0:w3544:string)  [unwired: 3 in]
                                n1857 = Number To Engineering String(4:w3522) -> (0:w3527:string)  [unwired: 3 in]
                                n1858 = Greater Or Equal?(x=w3551, y=w3536) -> (x >= y?=w3552:bool)
                                n1859 = Number To Decimal String(number=w3539) -> (decimal integer string=w3545:string)  [unwired: 1 in]
                                n1860 = Concatenate Strings(w3545, w3531, w3544, w3531, w3543, w3531, w3542, w3531, w3541, w3531, w3527, w3531, w3528, w3531, w3529) -> (w3546:string)
                                n1861 = Spreadsheet String To Array(delimiter (Tab)=w3531, format string="%s", spreadsheet string=w3546, array type (2D Dbl)=string[] []) -> (array=w3547:string[])
                                n1862 = Insert Into Array(array=w3532, index (row)=w3537, new element=w3547) -> (w3538:string[][])  [unwired: 1 in]
                                }
                                n1863 = Insert Into Array(array=w3487, new element=w3488) -> (w3504:string[][])  [unwired: 2 in]
                                n1864 = Equal?(x=w3492, y=w3486) -> (x = y?=w3509:bool)
                                n1865 = Index Array(array=w3504, index (col)=w3503) -> (element=w3501:string[])  [unwired: 1 in]
                                n1866 = Fract/Exp String To Number(string=w3501) -> (number=w3499:dbl[])  [unwired: 3 in, 1 out]
                                n1867 = call "Convert to Dynamic Data14"("Array"=w3499) -> ("Dynamic Data Type"=w3498:dynamicdata)  [unwired: 3 in]
                                n1868 = property on="PULSE DATA SHEET" class="Tbl (strict)"("Value"=w3504, "Edit Position"=w3491) -> ()  [unwired: 2 in, 2 out]
                                n1869 = Index Array(array=w3504, index (col)=w3502) -> (element=w3500:string[])  [unwired: 1 in]
                                n1870 = Fract/Exp String To Number(string=w3500) -> (number=w3497:dbl[])  [unwired: 3 in, 1 out]
                                n1871 = call "Convert to Dynamic Data15"("Array"=w3497) -> ("Dynamic Data Type"=w3496:dynamicdata)  [unwired: 3 in]
                                n1872 = call "Build XY Graph7"("Y Input"=w3496, "X Input"=w3498) -> ("XY Graph"=w3512:cluster{"Y":dbl[], "Y":dbl[]}[])  [unwired: 8 in, 1 out]
                                n1873 = property on="Pulsed IV Graph" class="XYGraph (strict)"("Value"=w3512) -> ()  [unwired: 2 in, 2 out]
                                n1874 = case shown="Error" w3514 {
                                tunnel: [w3562 TRUE] -> w3513
                                tunnel: w3493 -> [w3562 _]
                                frame No Error {
                                }
                                frame Error {
                                n1875 = call "RUN PULSE ERROR5"() -> ()  [unwired: 10 in, 2 out]
                                }
                                }
                                n1876 = Or(x=w3513, y=w3509) -> (x .or. y?=w3510:bool)
                                n1877 = Increment(x=w3486) -> (x+1=w3485:dbl)
                                }
                                }
                                n1878 = flat-sequence {
                                tunnel: w3429 -> [w3434]
                                tunnel: w3430 -> [w3435]
                                tunnel: [w3435] -> w3432
                                tunnel: [w3434] -> w3431
                                tunnel: [w3457] -> w3428
                                tunnel: [w3459] -> w3420
                                tunnel: [w3458] -> w3419
                                tunnel: w3432 -> [w3456]
                                tunnel: w3431 -> [w3451]
                                tunnel: w3415 -> [w3440]
                                frame #0 {
                                n1879 = Wait (ms)(milliseconds to wait=u32 2000) -> ()  [unwired: 1 out]
                                }
                                frame #1 {
                                n1880 = call "VISAreadWrite.vi"("GPIB INDEX Array"=i32[] [4], "GPIB ARRAY"=w3451, "VISA REFERENCE"=w3456) -> ("error out 15"=w3454:errorcluster, "Read Buffer Array"=w3452:string[])  [unwired: 1 in]
                                n1881 = Index Array(array=w3452, index=1) -> (element=w3442:string)
                                n1882 = Number To Decimal String(number=w3440) -> (decimal integer string=w3443:string)  [unwired: 1 in]
                                n1883 = Insert Into Array(array=string[] [] ("Replace Array"), index=0, new element=w3443) -> (w3447:string[])
                                n1884 = Decimal String To Number(string=w3442) -> (number=w3441:i32)  [unwired: 2 in, 1 out]
                                n1885 = Subtract(x=w3441, y=w3440) -> (x-y=w3438:dbl)
                                n1886 = Round To Nearest(number=w3438) -> (nearest integer value=w3436:dbl)
                                n1887 = Less Or Equal To 0?(x=w3436) -> (x <= 0?=w3437:bool)
                                n1888 = Number To Decimal String(number=w3436) -> (decimal integer string=w3439:string)  [unwired: 1 in]
